vi "Lighthouse Monitoring & Control System 7.vi"() -> ()   [LabVIEW 2012]
uses:
  <vilib>/DAQmx/read.llb/DAQmx Read (Counter DBL 1Chan 1Samp).vi
  <vilib>/DAQmx/write.llb/DAQmx Write (Digital U8 1Chan 1Samp).vi
  <vilib>/DAQmx/write.llb/DAQmx Write (Digital 1D Bool NChan 1Samp 1Line).vi
  <vilib>/DAQmx/write.llb/DAQmx Write (Analog DBL 1Chan 1Samp).vi
  <vilib>/DAQmx/read.llb/DAQmx Read (Analog DBL 1Chan 1Samp).vi
  <vilib>/DAQmx/create/channels.llb/DAQmx Create Channel (CI-Count Edges).vi
  <vilib>/DAQmx/create/channels.llb/DAQmx Create Channel (DO-Digital Output).vi
  <vilib>/DAQmx/create/channels.llb/DAQmx Create Channel (AI-Voltage-Basic).vi
  <vilib>/DAQmx/create/channels.llb/DAQmx Create Channel (AO-Voltage-Basic).vi
  <vilib>/DAQmx/miscellaneous.llb/DAQmx Fill In Error Info.vi
panel:
  out "Array":bool[](array[boolean])
  out "Data to Write":u32=255 format="%x"
  out "Voltage":dbl
  in  "?":bool
  out "Slot Count":dbl
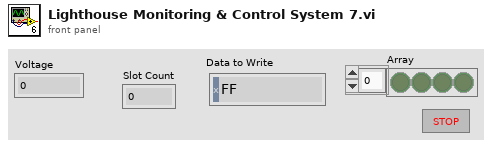
[diagram p1: front panel]
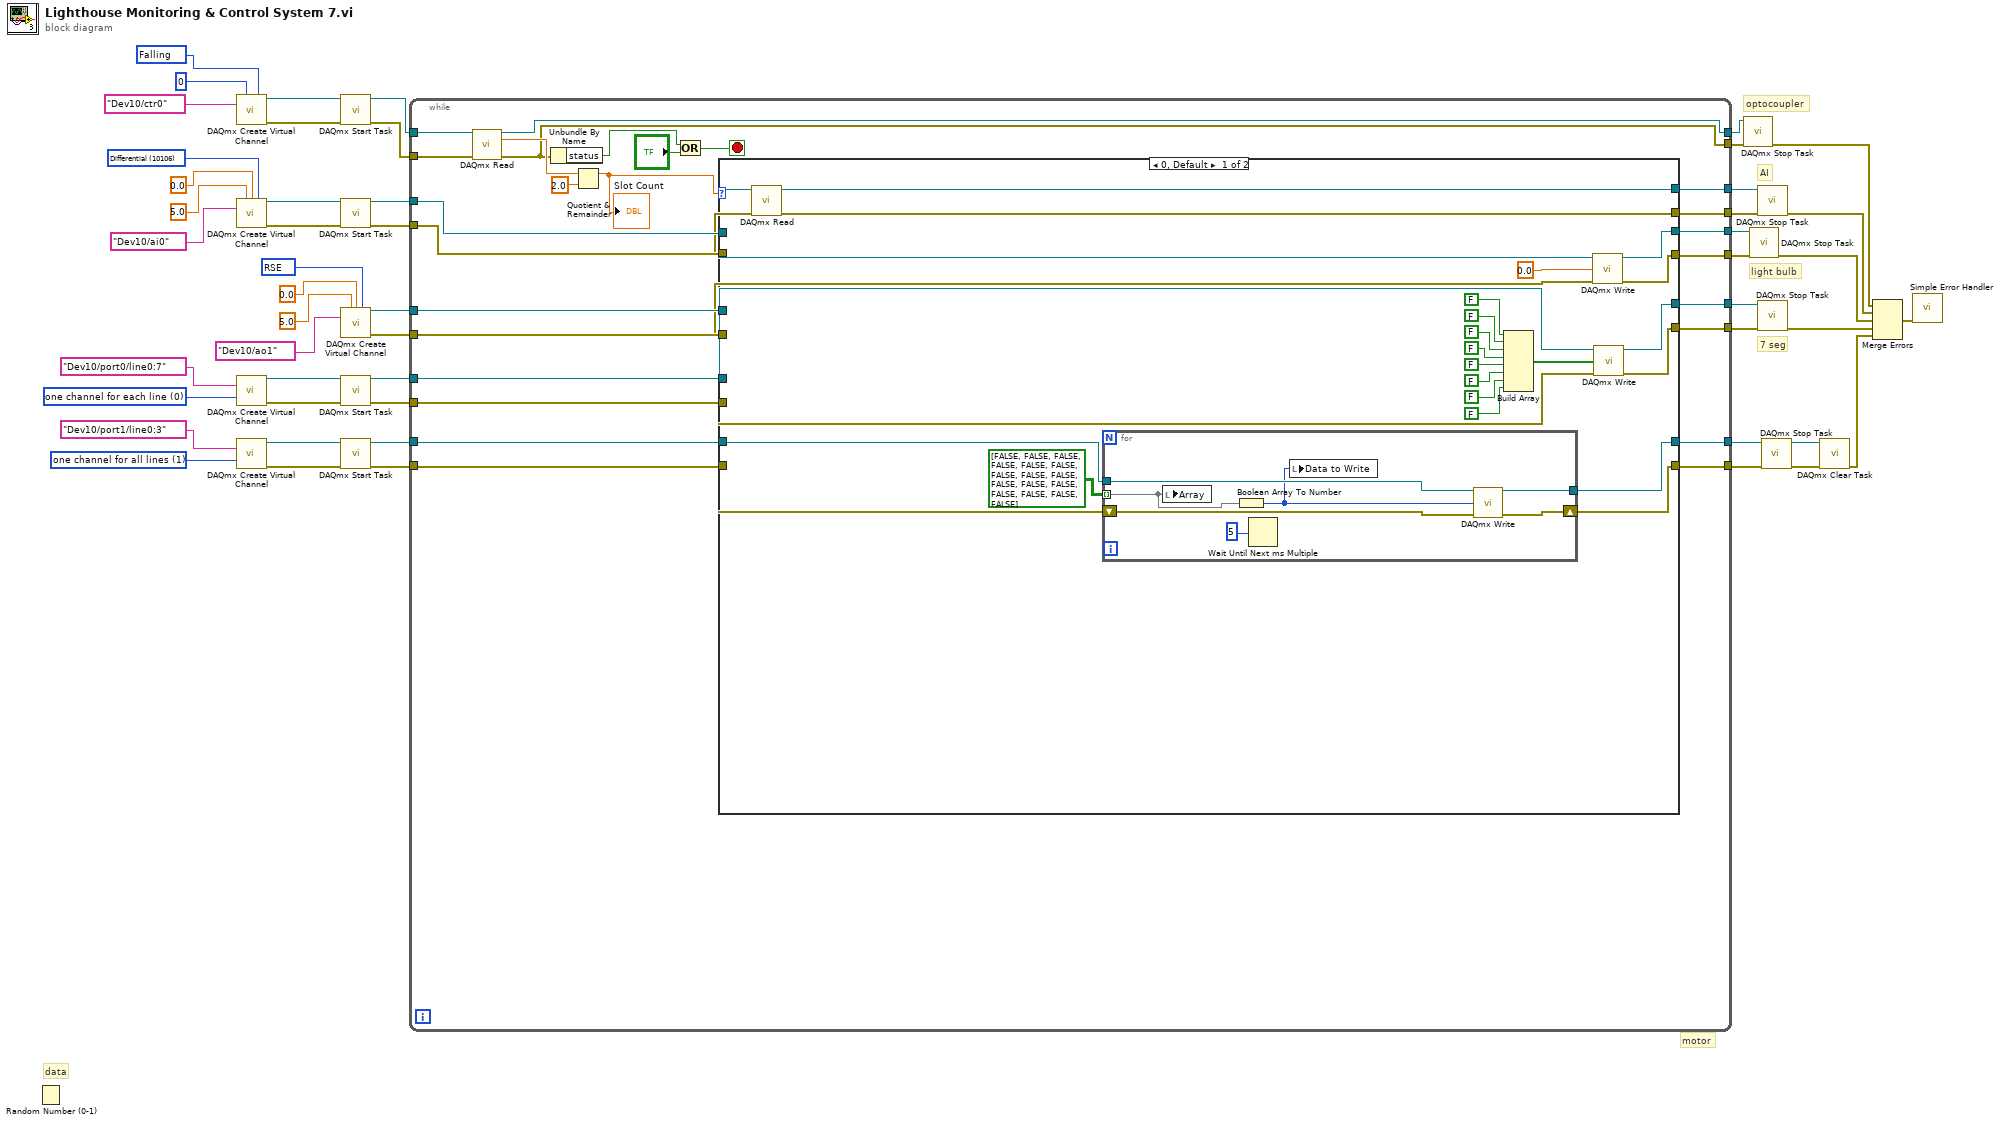
[diagram p0: block diagram]
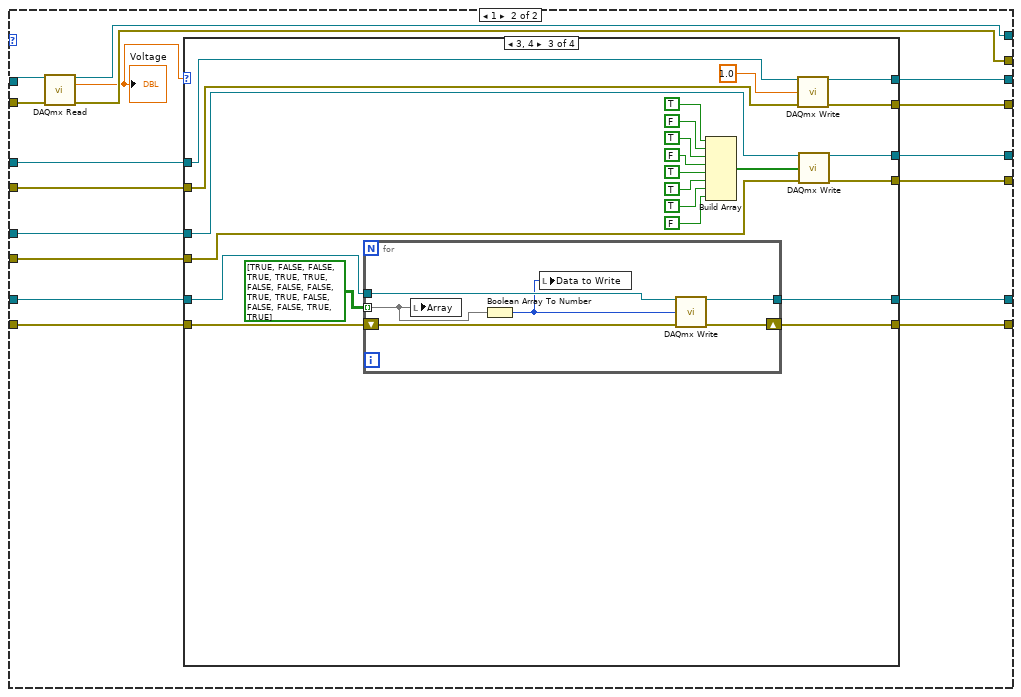
[diagram p2: hidden frame]
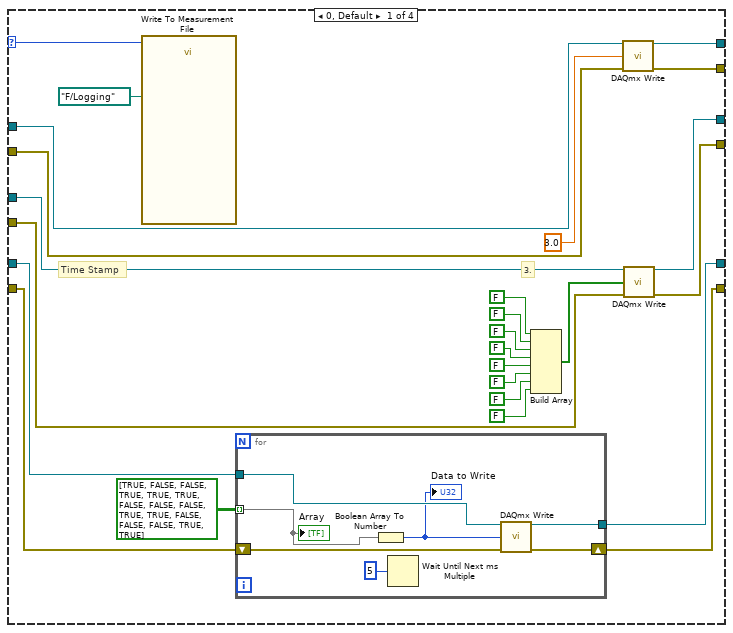
[diagram p3: hidden frame]
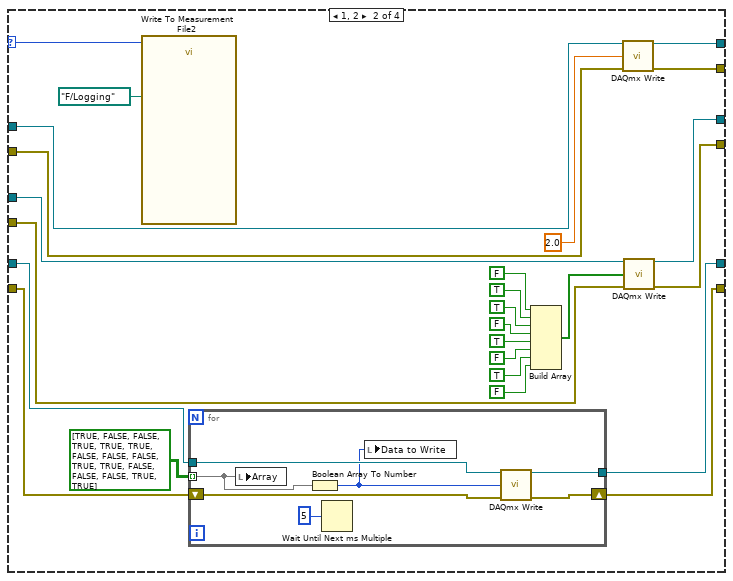
[diagram p4: hidden frame]
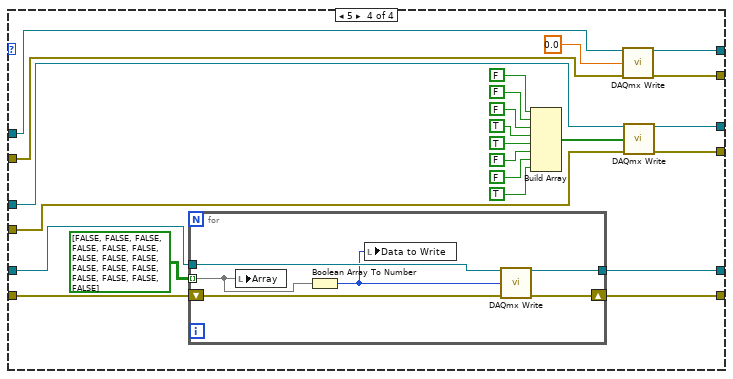
[diagram p5: hidden frame]
diagram:
  w11 = 1 items=["one channel for each line", "one channel for all lines"] ("line grouping")
  w38 = 0 items=["one channel for each line", "one channel for all lines"] ("line grouping")
  w41 = 10083 items=["Default"=-1, "RSE"=10083, "Differential"=10106, "Pseudodifferential"=12529] ("output terminal configuration")
  w44 = 10106 items=["default"=-1, "RSE"=10083, "NRSE"=10078, "Differential"=10106, "Pseudodifferential"=12529] ("input terminal configuration")
  w51 = 10171 items=["Rising"=10280, "Falling"=10171] ("edge")
  # "data"
  # "motor"
  # "7 seg"
  # "AI"
  # "light bulb"
  # "optocoupler"
  n1 = Random Number (0-1)() -> ()  [unwired: 1 out]
  n2 = call-poly <vilib>:"DAQmx Create Virtual Channel.vi"("initial count"=u32 0, "edge"=w51, "counter"=tag "Dev10/ctr0") -> ("task out"=w50:refnum<k21>, "error out"=w49:errorcluster)  [unwired: 11 in]
  n3 = call-poly <vilib>:"DAQmx Create Virtual Channel.vi"("maximum value"=5.0, "minimum value"=0.0, "input terminal configuration"=w44, "physical channels"=tag "Dev10/ai0") -> ("task out"=w42:refnum<k21>, "error out"=w43:errorcluster)  [unwired: 10 in]
  n4 = call-poly <vilib>:"DAQmx Create Virtual Channel.vi"("lines"=tag "Dev10/port0/line0:7", "line grouping"=w38) -> ("task out"=w37:refnum<k21>, "error out"=w36:errorcluster)  [unwired: 12 in]
  n5 = call-poly <vilib>:"DAQmx Create Virtual Channel.vi"("lines"=tag "Dev10/port1/line0:3", "line grouping"=w11) -> ("task out"=w10:refnum<k21>, "error out"=w9:errorcluster)  [unwired: 12 in]
  n6 = call <vilib>:"DAQmx Start Task.vi"("task/channels in"=w50, "error in"=w49) -> ("task out"=w46:refnum<k21>, "error out"=w45:errorcluster)  [unwired: 12 in]
  n7 = call <vilib>:"DAQmx Start Task.vi"("task/channels in"=w42, "error in"=w43) -> ("task out"=w32:refnum<k21>, "error out"=w31:errorcluster)  [unwired: 12 in]
  n8 = call-poly <vilib>:"DAQmx Create Virtual Channel.vi"("maximum value"=5.0, "minimum value"=0.0, "output terminal configuration"=w41, "physical channels"=tag "Dev10/ao1") -> ("task out"=w30:refnum<k21>, "error out"=w29:errorcluster)  [unwired: 10 in]
  n9 = call <vilib>:"DAQmx Start Task.vi"("task/channels in"=w37, "error in"=w36) -> ("task out"=w28:refnum<k21>, "error out"=w27:errorcluster)  [unwired: 12 in]
  n10 = call <vilib>:"DAQmx Start Task.vi"("task/channels in"=w10, "error in"=w9) -> ("task out"=w8:refnum<k21>, "error out"=w7:errorcluster)  [unwired: 12 in]
  n11 = while {
    tunnel: w46 -> [w77]
    tunnel: w45 -> [w76]
    tunnel: [w64] -> w34
    tunnel: w32 -> [w70]
    tunnel: w31 -> [w69]
    tunnel: w30 -> [w68]
    tunnel: w29 -> [w67]
    tunnel: w28 -> [w66]
    tunnel: w27 -> [w65]
    tunnel: [w63] -> w22
    tunnel: [w62] -> w21
    tunnel: [w61] -> w20
    tunnel: [w60] -> w19
    tunnel: [w59] -> w18
    tunnel: [w58] -> w17
    tunnel: [w57] -> w16
    tunnel: w8 -> [w56]
    tunnel: w7 -> [w55]
    tunnel: [w53] -> w3
    tunnel: [w54] -> w2
    stop <- w73 stop-if-true
    n12 = call-poly <vilib>:"DAQmx Read.vi"("task/channels in"=w77, "error in"=w76) -> ("task out"=w64:refnum<k21>, "data"=w75:dbl, "error out"=w63:errorcluster)  [unwired: 11 in]
    n13 = Unbundle By Name(w63) -> ("status"=w72:bool)
    n14 = Quotient & Remainder(x=w75, y=2.0) -> (x-y*floor(x/y)=w52:dbl)  [unwired: 1 out]
    "Slot Count" <- w52
    n15 = Or(x=w72, y="?") -> (x .or. y?=w73:bool)
    n16 = case shown="0, Default" w52 {
      tunnel: w70 -> [w101 w128]
      tunnel: w69 -> [w100 w127]
      tunnel: w68 -> [w99 w126]
      tunnel: w67 -> [w98 w125]
      tunnel: w66 -> [w103 w124]
      tunnel: w65 -> [w102 w123]
      tunnel: [w95 w122] -> w58
      tunnel: [w96 w121] -> w62
      tunnel: [w97 w120] -> w61
      tunnel: [w92 w119] -> w60
      tunnel: [w93 w118] -> w59
      tunnel: [w94 w117] -> w57
      tunnel: w56 -> [w81 w116]
      tunnel: w55 -> [w80 w115]
      tunnel: [w78 w113] -> w54
      tunnel: [w79 w114] -> w53
      frame 0, Default {
        n17 = call-poly <vilib>:"DAQmx Read.vi"("task/channels in"=w101, "error in"=w100) -> ("task out"=w94:refnum<k21>, "error out"=w97:errorcluster)  [unwired: 11 in, 1 out]
        n18 = for {
          tunnel: w81 -> [w110]
          tunnel: [w109] -> w79
          shift-right: [w107] -> w78
          shift-left: w80 -> [w111]
          tunnel: bool[][] [[FALSE, FALSE, FALSE, FALSE], [FALSE, FALSE, FALSE, FALSE], [FALSE, FALSE, FALSE, FALSE], [FALSE, FALSE, FALSE, FALSE]] -> [w105] mode=indexing
          n19 = local write "Array"(w105) -> ()
          n20 = Boolean Array To Number(Boolean array=w105) -> (number=w106:u32)
          n21 = Wait Until Next ms Multiple(millisecond multiple=5) -> ()  [unwired: 1 out]
          n22 = local write "Data to Write"(w106) -> ()
          n23 = call-poly <vilib>:"DAQmx Write.vi"("task/channels in"=w110, "data"=w106, "error in"=w111) -> ("task out"=w109:refnum<k21>, "error out"=w107:errorcluster)  [unwired: 10 in, 1 out]
        }
        n24 = Build Array(FALSE, FALSE, FALSE, FALSE, FALSE, FALSE, FALSE, FALSE) -> (w83:bool[])
        n25 = call-poly <vilib>:"DAQmx Write.vi"("task/channels in"=w99, "data"=0.0, "error in"=w98) -> ("task out"=w95:refnum<k21>, "error out"=w96:errorcluster)  [unwired: 10 in, 1 out]
        n26 = call-poly <vilib>:"DAQmx Write.vi"("task/channels in"=w103, "data"=w83, "error in"=w102) -> ("task out"=w93:refnum<k21>, "error out"=w92:errorcluster)  [unwired: 10 in, 1 out]
      }
      frame 1 {
        n27 = call-poly <vilib>:"DAQmx Read.vi"("task/channels in"=w128, "error in"=w127) -> ("task out"=w117:refnum<k21>, "data"=w112:dbl, "error out"=w120:errorcluster)  [unwired: 11 in]
        "Voltage" <- w112
        n28 = case shown="3, 4" w112 {
          selector: w112 -> [w129 w161 _ _]
          tunnel: w126 -> [w139 w175 w205 w234]
          tunnel: w125 -> [w138 w174 w204 w233]
          tunnel: [w143 w173 w203 w232] -> w122
          tunnel: [w142 w172 w202 w231] -> w121
          tunnel: [w141 w171 w201 w230] -> w118
          tunnel: [w140 w170 w200 w229] -> w119
          tunnel: w124 -> [w137 w169 w199 w228]
          tunnel: w123 -> [w136 w168 w198 w227]
          tunnel: w116 -> [w135 w166 w196 w225]
          tunnel: w115 -> [w134 w165 w195 w224]
          tunnel: [w133 w164 w194 w223] -> w114
          tunnel: [w132 w163 w193 w222] -> w113
          frame 0, Default {
            # "3."
            # "Time Stamp"
            n29 = call "Write To Measurement File"("Signals"=w129, "Filename"=path "F:/Logging") -> ()  [unwired: 15 in, 3 out]
            n30 = for {
              tunnel: w135 -> [w159]
              tunnel: [w158] -> w133
              shift-right: [w157] -> w132
              shift-left: w134 -> [w160]
              tunnel: bool[][] [[TRUE, FALSE, FALSE, TRUE], [TRUE, TRUE, FALSE, FALSE], [FALSE, TRUE, TRUE, FALSE], [FALSE, FALSE, TRUE, TRUE]] -> [w155] mode=indexing
              n31 = Boolean Array To Number(Boolean array=w155) -> (number=w156:u32)
              "Data to Write" <- w156
              n32 = Wait Until Next ms Multiple(millisecond multiple=u32 5) -> ()  [unwired: 1 out]
              n33 = call-poly <vilib>:"DAQmx Write.vi"("task/channels in"=w159, "data"=w156, "error in"=w160) -> ("task out"=w158:refnum<k21>, "error out"=w157:errorcluster)  [unwired: 10 in, 1 out]
              "Array" <- w155
            }
            n34 = Build Array(FALSE, FALSE, FALSE, FALSE, FALSE, FALSE, FALSE, FALSE) -> (w144:bool[])
            n35 = call-poly <vilib>:"DAQmx Write.vi"("task/channels in"=w139, "data"=3.0, "error in"=w138) -> ("task out"=w143:refnum<k21>, "error out"=w142:errorcluster)  [unwired: 10 in, 1 out]
            n36 = call-poly <vilib>:"DAQmx Write.vi"("task/channels in"=w137, "data"=w144, "error in"=w136) -> ("task out"=w141:refnum<k21>, "error out"=w140:errorcluster)  [unwired: 10 in, 1 out]
          }
          frame 1, 2 {
            n37 = call "Write To Measurement File2"("Signals"=w161, "Filename"=path "F:/Logging") -> ()  [unwired: 15 in, 3 out]
            n38 = for {
              tunnel: w166 -> [w187]
              tunnel: [w191] -> w164
              shift-right: [w190] -> w163
              shift-left: w165 -> [w192]
              tunnel: bool[][] [[TRUE, FALSE, FALSE, TRUE], [TRUE, TRUE, FALSE, FALSE], [FALSE, TRUE, TRUE, FALSE], [FALSE, FALSE, TRUE, TRUE]] -> [w188] mode=indexing
              n39 = local write "Array"(w188) -> ()
              n40 = Boolean Array To Number(Boolean array=w188) -> (number=w186:u32)
              n41 = Wait Until Next ms Multiple(millisecond multiple=u32 5) -> ()  [unwired: 1 out]
              n42 = local write "Data to Write"(w186) -> ()
              n43 = call-poly <vilib>:"DAQmx Write.vi"("task/channels in"=w187, "data"=w186, "error in"=w192) -> ("task out"=w191:refnum<k21>, "error out"=w190:errorcluster)  [unwired: 10 in, 1 out]
            }
            n44 = Build Array(FALSE, TRUE, TRUE, FALSE, TRUE, FALSE, TRUE, FALSE) -> (w176:bool[])
            n45 = call-poly <vilib>:"DAQmx Write.vi"("task/channels in"=w175, "data"=2.0, "error in"=w174) -> ("task out"=w173:refnum<k21>, "error out"=w172:errorcluster)  [unwired: 10 in, 1 out]
            n46 = call-poly <vilib>:"DAQmx Write.vi"("task/channels in"=w169, "data"=w176, "error in"=w168) -> ("task out"=w171:refnum<k21>, "error out"=w170:errorcluster)  [unwired: 10 in, 1 out]
          }
          frame 3, 4 {
            n47 = for {
              tunnel: w196 -> [w220]
              tunnel: [w219] -> w194
              shift-right: [w218] -> w193
              shift-left: w195 -> [w221]
              tunnel: bool[][] [[TRUE, FALSE, FALSE, TRUE], [TRUE, TRUE, FALSE, FALSE], [FALSE, TRUE, TRUE, FALSE], [FALSE, FALSE, TRUE, TRUE]] -> [w217] mode=indexing
              n48 = local write "Array"(w217) -> ()
              n49 = Boolean Array To Number(Boolean array=w217) -> (number=w216:u32)
              n50 = local write "Data to Write"(w216) -> ()
              n51 = call-poly <vilib>:"DAQmx Write.vi"("task/channels in"=w220, "data"=w216, "error in"=w221) -> ("task out"=w219:refnum<k21>, "error out"=w218:errorcluster)  [unwired: 10 in, 1 out]
            }
            n52 = Build Array(TRUE, FALSE, TRUE, FALSE, TRUE, TRUE, TRUE, FALSE) -> (w206:bool[])
            n53 = call-poly <vilib>:"DAQmx Write.vi"("task/channels in"=w205, "data"=1.0, "error in"=w204) -> ("task out"=w203:refnum<k21>, "error out"=w202:errorcluster)  [unwired: 10 in, 1 out]
            n54 = call-poly <vilib>:"DAQmx Write.vi"("task/channels in"=w199, "data"=w206, "error in"=w198) -> ("task out"=w201:refnum<k21>, "error out"=w200:errorcluster)  [unwired: 10 in, 1 out]
          }
          frame 5 {
            n55 = for {
              tunnel: w225 -> [w249]
              tunnel: [w248] -> w223
              shift-right: [w247] -> w222
              shift-left: w224 -> [w250]
              tunnel: bool[][] [[FALSE, FALSE, FALSE, FALSE], [FALSE, FALSE, FALSE, FALSE], [FALSE, FALSE, FALSE, FALSE], [FALSE, FALSE, FALSE, FALSE]] -> [w246] mode=indexing
              n56 = local write "Array"(w246) -> ()
              n57 = Boolean Array To Number(Boolean array=w246) -> (number=w245:u32)
              n58 = local write "Data to Write"(w245) -> ()
              n59 = call-poly <vilib>:"DAQmx Write.vi"("task/channels in"=w249, "data"=w245, "error in"=w250) -> ("task out"=w248:refnum<k21>, "error out"=w247:errorcluster)  [unwired: 10 in, 1 out]
            }
            n60 = Build Array(FALSE, FALSE, FALSE, TRUE, TRUE, FALSE, FALSE, TRUE) -> (w235:bool[])
            n61 = call-poly <vilib>:"DAQmx Write.vi"("task/channels in"=w234, "data"=0.0, "error in"=w233) -> ("task out"=w232:refnum<k21>, "error out"=w231:errorcluster)  [unwired: 10 in, 1 out]
            n62 = call-poly <vilib>:"DAQmx Write.vi"("task/channels in"=w228, "data"=w235, "error in"=w227) -> ("task out"=w230:refnum<k21>, "error out"=w229:errorcluster)  [unwired: 10 in, 1 out]
          }
        }
      }
    }
  }
  n63 = call <vilib>:"DAQmx Stop Task.vi"("task/channels in"=w34, "error in"=w22) -> ("error out"=w33:errorcluster)  [unwired: 12 in, 1 out]
  n64 = call <vilib>:"DAQmx Stop Task.vi"("task/channels in"=w17, "error in"=w21) -> ("error out"=w25:errorcluster)  [unwired: 12 in, 1 out]
  n65 = call <vilib>:"DAQmx Stop Task.vi"("task/channels in"=w16, "error in"=w20) -> ("error out"=w26:errorcluster)  [unwired: 12 in, 1 out]
  n66 = call <vilib>:"DAQmx Stop Task.vi"("task/channels in"=w18, "error in"=w19) -> ("error out"=w24:errorcluster)  [unwired: 12 in, 1 out]
  n67 = call <vilib>:"DAQmx Stop Task.vi"("task/channels in"=w3, "error in"=w2) -> ("task out"=w6:refnum<k21>, "error out"=w5:errorcluster)  [unwired: 12 in]
  n68 = call <vilib>:"DAQmx Clear Task.vi"("task in"=w6, "error in"=w5) -> ("error out"=w4:errorcluster)  [unwired: 13 in]
  n69 = Merge Errors(w33, w26, w25, w24, w4) -> (w23:errorcluster)
  n70 = call <vilib>:"Simple Error Handler.vi"("error in (no error)"=w23) -> ()  [unwired: 4 in, 5 out]
